vi "FromEnergy.vi"(0 "A":dbl, 1 "Z":dbl, 2 "E (MeV)":dbl, 3 "Rm":dbl, 4 "UECR":dbl, 5 "HARM":dbl=3.0, 6 "Rextr":dbl=1.78) -> (7 "Uinfl":dbl, 9 "Ubender":dbl, 11 "UIAT":dbl, 12 "Udef":dbl, 13 "Uinj":dbl, 14 "A/Z":dbl, 15 "F":dbl, 16 "MeV/u":dbl, 17 "B0(kGs)":dbl, 18 "B0(T)":dbl, 19 "Im":dbl)   [LabVIEW 2018, in "Class 2.lvclass"]
uses:
  Class 2.lvclass
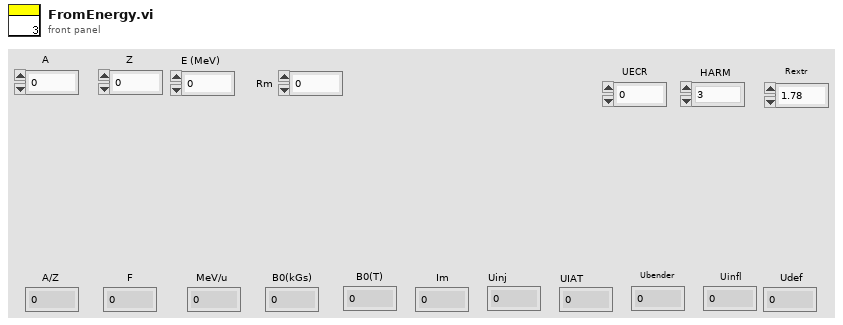
[diagram p1: front panel]
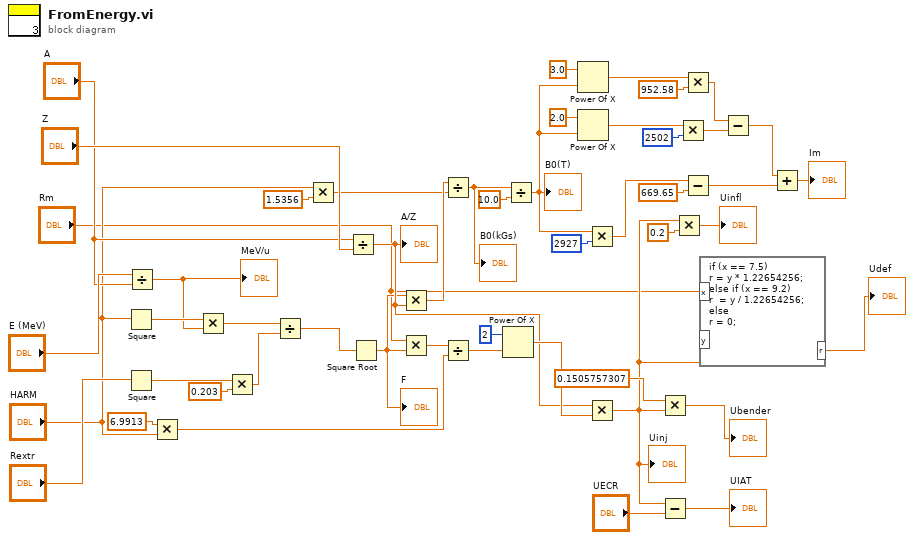
[diagram p0: block diagram]
diagram:
  n1 = Square(x="HARM") -> (x^2=w46:dbl)
  n2 = Square(x="Rextr") -> (x^2=w44:dbl)
  n3 = Divide(x="E (MeV)", y="A") -> (x/y=w5:dbl)
  "MeV/u" <- w5
  n4 = Multiply(x=6.9913, y="HARM") -> (x*y=w20:dbl)
  n5 = Multiply(x=w46, y=w5) -> (x*y=w42:dbl)
  n6 = Multiply(x=w44, y=0.203) -> (x*y=w41:dbl)
  n7 = Divide(x=w42, y=w41) -> (x/y=w40:dbl)
  n8 = Multiply(x="HARM", y=1.5356) -> (x*y=w37:dbl)
  n9 = Divide(x="A", y="Z") -> (x/y=w9:dbl)
  "A/Z" <- w9
  n10 = Square Root(x=w40) -> (sqrt(x)=w8:dbl)
  "F" <- w8
  n11 = Multiply(x=w8, y=w9) -> (x*y=w38:dbl)
  n12 = Multiply(x="Rm", y=w8) -> (x*y=w21:dbl)
  n13 = Divide(x=w38, y=w37) -> (x/y=w6:dbl)
  "B0(kGs)" <- w6
  n14 = Divide(x=w21, y=w20) -> (x/y=w19:dbl)
  n15 = Power Of X(1:w19, 2:2) -> (0:w17:dbl)
  n16 = Divide(x=w6, y=10.0) -> (x/y=w7:dbl)
  "B0(T)" <- w7
  n17 = Power Of X(1:w7, 2:3.0 ("y")) -> (0:w34:dbl)
  n18 = Power Of X(1:w7, 2:2.0 ("y")) -> (0:w32:dbl)
  n19 = Multiply(x=w7, y=2927) -> (x*y=w26:dbl)
  n20 = Multiply(x=w9, y=w17) -> (x*y=w3:dbl)
  "Uinj" <- w3
  n21 = Multiply(x=0.1505757307, y=w3) -> (x*y=→"Ubender":dbl)
  n22 = Subtract(x=w3, y="UECR") -> (x-y=→"UIAT":dbl)
  n23 = Multiply(x=w3, y=0.2) -> (x*y=→"Uinfl":dbl)
  n24 = Multiply(x=w32, y=2502) -> (x*y=w27:dbl)
  n25 = Multiply(x=w34, y=952.58) -> (x*y=w28:dbl)
  n26 = Subtract(x=w26, y=669.65) -> (x-y=w23:dbl)
  n27 = formula code="if (x == 7.5)\nr = y * 1.22654256;\nelse if (x == 9.2)\nr  = y / 1.22654256;\nelse\nr = 0;"("x"="Rm", "y"=w3) -> ("r"=→"Udef":dbl)
  n28 = Subtract(x=w28, y=w27) -> (x-y=w24:dbl)
  n29 = Add(x=w24, y=w23) -> (x+y=→"Im":dbl)
